vi "WPI_DMAChannelsGlobal.vi"(8 "Clear":bool, 9 "Start":bool, 10 "Channel":cluster{"Channel Type":T1, "Channel Number":u8}, 11 "Add":bool) -> (0 "Packed Bytes Per Sample":i32, 1 "Started":bool, 2 "Channels Out":T2(array[cluster]))   [LabVIEW 2017]
uses:
  <vilib>/Rock Robotics/WPI/DMA/WPI_DMAChannelTypeEnum.ctl
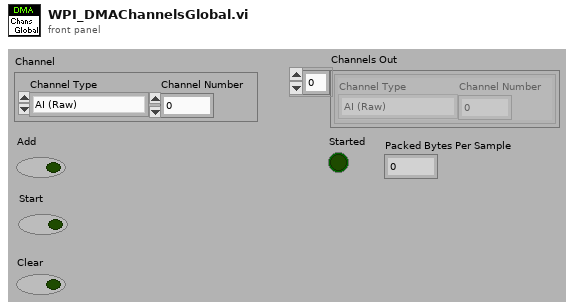
[diagram p1: front panel]
types:
  T1 = typedef "WPI_DMAChannelTypeEnum.ctl" = enum16{"AI (Raw)", "AI (Avg)", "Accumulator", "DI (Raw) Onboard", "DI (Filtered) Onboard", "DI (Raw) MXP", "DI (Filtered) MXP", "Analog Trigger", "Counter", "Counter (Timer)", "Encoder", "Encoder (Timer)", "Time Stamp"}
  T2 = cluster{"Channel Type":T1, "Channel Number":u8}[]
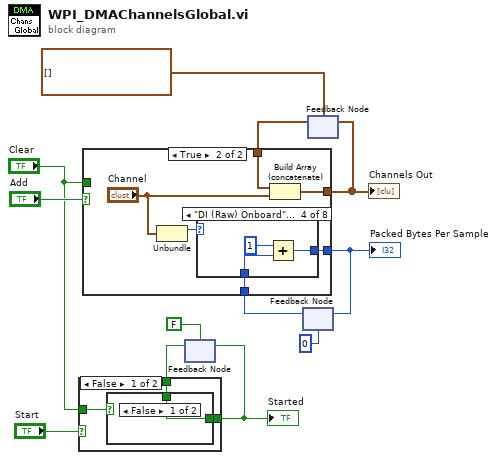
[diagram p0: block diagram]
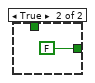
[diagram p2: hidden frame]
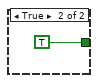
[diagram p3: hidden frame]
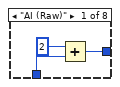
[diagram p6: hidden frame]
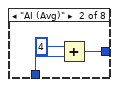
[diagram p7: hidden frame]
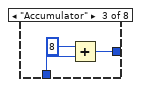
[diagram p8: hidden frame]
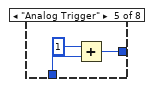
[diagram p9: hidden frame]
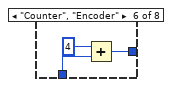
[diagram p10: hidden frame]
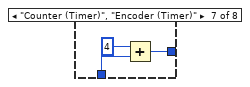
[diagram p11: hidden frame]
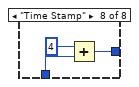
[diagram p12: hidden frame]
diagram:
  n1 = feedback #1(FALSE) -> (w5:bool)
  n2 = case shown="False" "Start" {
    tunnel: "Clear" -> [w15 _]
    tunnel: [w14 TRUE] -> w4
    tunnel: w5 -> [w13 _]
    frame False {
      n3 = case shown="False" w15 {
        tunnel: [w16 FALSE] -> w14
        tunnel: w13 -> [w16 _]
        frame False {
        }
        frame True {
        }
      }
    }
    frame True {
    }
  }
  "Started" <- w4
  n4 = feedback-in #1(w4) -> ()
  n5 = feedback #2(0) -> (w2:i32)
  n6 = feedback #3(T2 [] ("Channels")) -> (w10:T2)
  n7 = case shown="True" "Add" {
    tunnel: [w22 w30] -> w11
    tunnel: w10 -> [w21 w31]
    tunnel: "Clear" -> [w23 _]
    tunnel: w2 -> [w19 w27]
    tunnel: [w20 w26] -> w1
    frame False {
      n8 = case shown="False" w23 {
        tunnel: [w25 _] -> w22
        tunnel: w21 -> [w25 _]
        tunnel: [w24 _] -> w20
        tunnel: w19 -> [w24 _]
        frame False {
        }
        frame True {
        }
      }
    }
    frame True {
      n9 = Unbundle("Channel") -> ("Channel Type"=w28:T1)  [unwired: 1 out]
      n10 = case shown="\"DI (Raw) Onboard\"..\"DI (Filtered) MXP\"" w28 {
        tunnel: w27 -> [w34 w37 w40 w43 w46 w49 w52 w55]
        tunnel: [w32 w35 w38 w41 w44 w47 w50 w53] -> w26
        frame "AI (Raw)" {
          n11 = Add(x=2, y=w34) -> (x+y=w32:i32)
        }
        frame "AI (Avg)" {
          n12 = Add(x=4, y=w37) -> (x+y=w35:i32)
        }
        frame "Accumulator" {
          n13 = Add(x=8, y=w40) -> (x+y=w38:i32)
        }
        frame "DI (Raw) Onboard".."DI (Filtered) MXP" {
          n14 = Add(x=1, y=w43) -> (x+y=w41:i32)
        }
        frame "Analog Trigger" {
          n15 = Add(x=1, y=w46) -> (x+y=w44:i32)
        }
        frame "Counter", "Encoder" {
          n16 = Add(x=4, y=w49) -> (x+y=w47:i32)
        }
        frame "Counter (Timer)", "Encoder (Timer)" {
          n17 = Add(x=4, y=w52) -> (x+y=w50:i32)
        }
        frame "Time Stamp" {
          n18 = Add(x=4, y=w55) -> (x+y=w53:i32)
        }
      }
      n19 = Build Array (concatenate)(w31, "Channel") -> (w30:T2)
    }
  }
  "Channels Out" <- w11
  "Packed Bytes Per Sample" <- w1
  n20 = feedback-in #2(w1) -> ()
  n21 = feedback-in #3(w11) -> ()
